vi "Sieve of Eratosthenes LV12 - NI Verified.vi"(11 "Final number":i32) -> (1 "size(s)":i32, 2 "Prime numbers":u32[](array[numeric]))   [LabVIEW 2025]
panel:
  # "Overview:  Coding that exemplifies the implementation of the sieve of Eratosthenes algorithm in LabVIEW.\nRequirements: LabVIEW 2012 or compatible\nInstructions:\n1. Select a number to limit the search\n2. Run the VI"
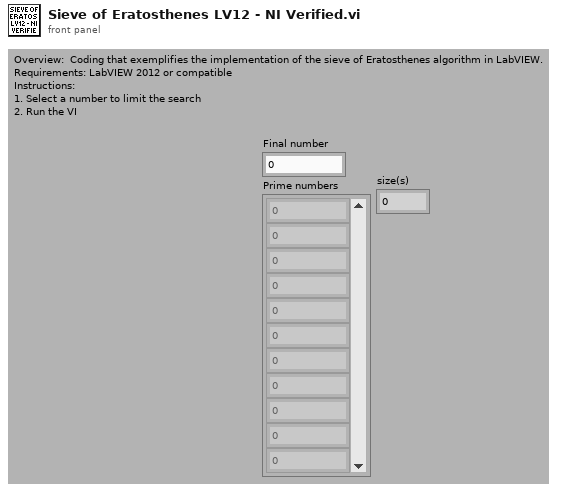
[diagram p1: front panel]
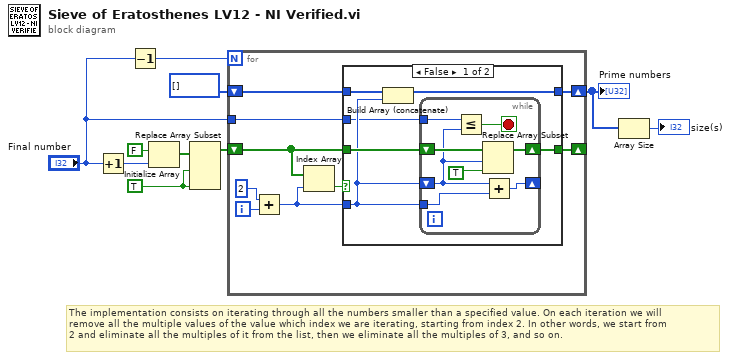
[diagram p0: block diagram]
diagram:
  w8 = TRUE
  # "The implementation consists on iterating through all the numbers smaller than a specified value. On each iteration we will\nremove all the multiple values of the value which index we are iterating, starting from index 2. In other words, we start from \n2 and eliminate all the multiples of it from the list, then we eliminate all the multiples of 3, and so on."
  n1 = Increment(x="Final number") -> (x+1=w5:i32)
  n2 = Decrement(x="Final number") -> (x-1=w4:i32)
  n3 = Initialize Array(FALSE, w5) -> (w9:bool[])
  n4 = Replace Array Subset(array=w9, new element #1=w8, new element #2=w8) -> (w7:bool[])  [unwired: 2 in]
  n5 = for {
    N: w4 -> [_]
    shift-right: [w14] -> w2
    shift-left: u32[] [] -> [w15]
    shift-right: [w13] -> _
    shift-left: w7 -> [w16]
    tunnel: "Final number" -> [w11]
    i -> [w19]
    n6 = Add(x=2, y=w19) -> (x+y=w12:i32)
    n7 = Index Array(array=w16, index=w12) -> (element=w17:bool)
    n8 = case shown="False" w17 {
      tunnel: w12 -> [w23 _]
      tunnel: w16 -> [w25 w35]
      tunnel: w15 -> [w24 w34]
      tunnel: [w22 w34] -> w14
      tunnel: [w21 w35] -> w13
      tunnel: w11 -> [w20 _]
      frame False {
        n9 = Build Array (concatenate)(w24, w23) -> (w22:u32[])
        n10 = while {
          shift-right: [w33] -> _
          shift-left: w23 -> [w28]
          tunnel: w23 -> [w32]
          shift-right: [w29] -> w21
          shift-left: w25 -> [w31]
          tunnel: w20 -> [w26]
          stop <- w27 stop-if-true
          n11 = Less Or Equal?(x=w26, y=w28) -> (x <= y?=w27:bool)
          n12 = Replace Array Subset(array=w31, new element=TRUE ("new element/subarray"), index=w28) -> (w29:bool[])
          n13 = Add(x=w28, y=w32) -> (x+y=w33:i32)
        }
      }
      frame True {
      }
    }
  }
  "Prime numbers" <- w2
  n14 = Array Size(array=w2) -> (size(s)=→"size(s)":i32)
